vi "CodigoLabView 3.vi"() -> (11 "Releb 2":bool)   [LabVIEW 2025]
uses:
  <vilib>/Utility/NIReport.llb/Report Type.ctl
  <vilib>/Instr/_visa.llb/VISA Configure Serial Port (Instr).vi
  <vilib>/addons/_office/excel.llb/Excel Easy Table (str).vi
  <vilib>/Utility/NIReport.llb/NI_report.lvclass
  <vilib>/Utility/NIReport.llb/NI_ReportGenerationCore.lvlib
  <vilib>/addons/_office/NI_ReportGenerationToolkit.lvlib
  <vilib>/Utility/NIReport.llb/Excel/NI_Excel.lvclass
panel:
  out "Releb 4":bool
  out "Relea 4":bool
  out "Rele 4":bool
  out "Boolean 4":bool
  out "Estado 4":string
  in  "Relé N°4":bool
  out "Potencia 4":string
  out "Releb 3":bool
  out "Relea 3":bool
  out "Rele 3":bool
  out "Boolean 3":bool
  out "Estado 3":string
  out "Potencia 3":string
  in  "Relé N°3":bool
  out "Relea 2":bool
  out "Rele 2":bool
  out "Boolean 2":bool
  out "Estado 2":string
  out "Potencia 2":string
  in  "Relé N°2":bool
  out "Releb 1":bool
  out "Relea 1":bool
  out "Rele 1":bool
  out "Boolean":bool
  out "Estado 1":string
  out "Potencia 1":string
  in  "Relé N°1":bool
  in  "template (empty)":path
  out "Tensión":string
  in  "VISA resource name":refnum<visa-resource-name>
  in  "stop":bool
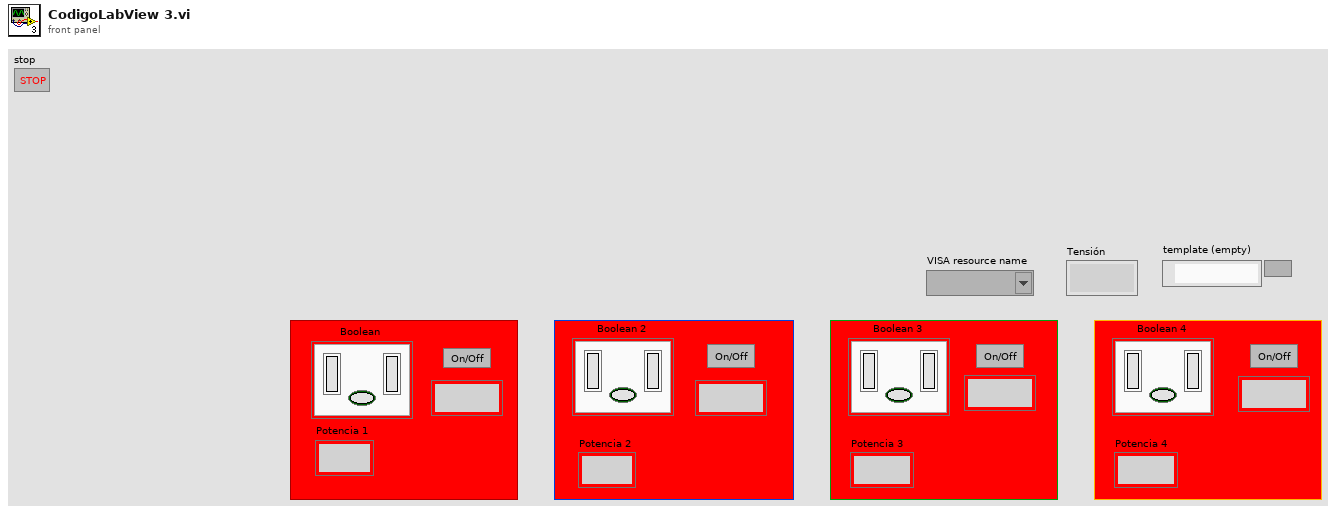
[diagram p1: front panel]
types:
  T1 = cluster{"W1":string, "W2":string, "W3":string, "W4":string, "V":string}
  T2 = typedef "NI_ReportGenerationCore.lvlib/Report Type.ctl" = enum16{"HTML", "Word", "Excel"}
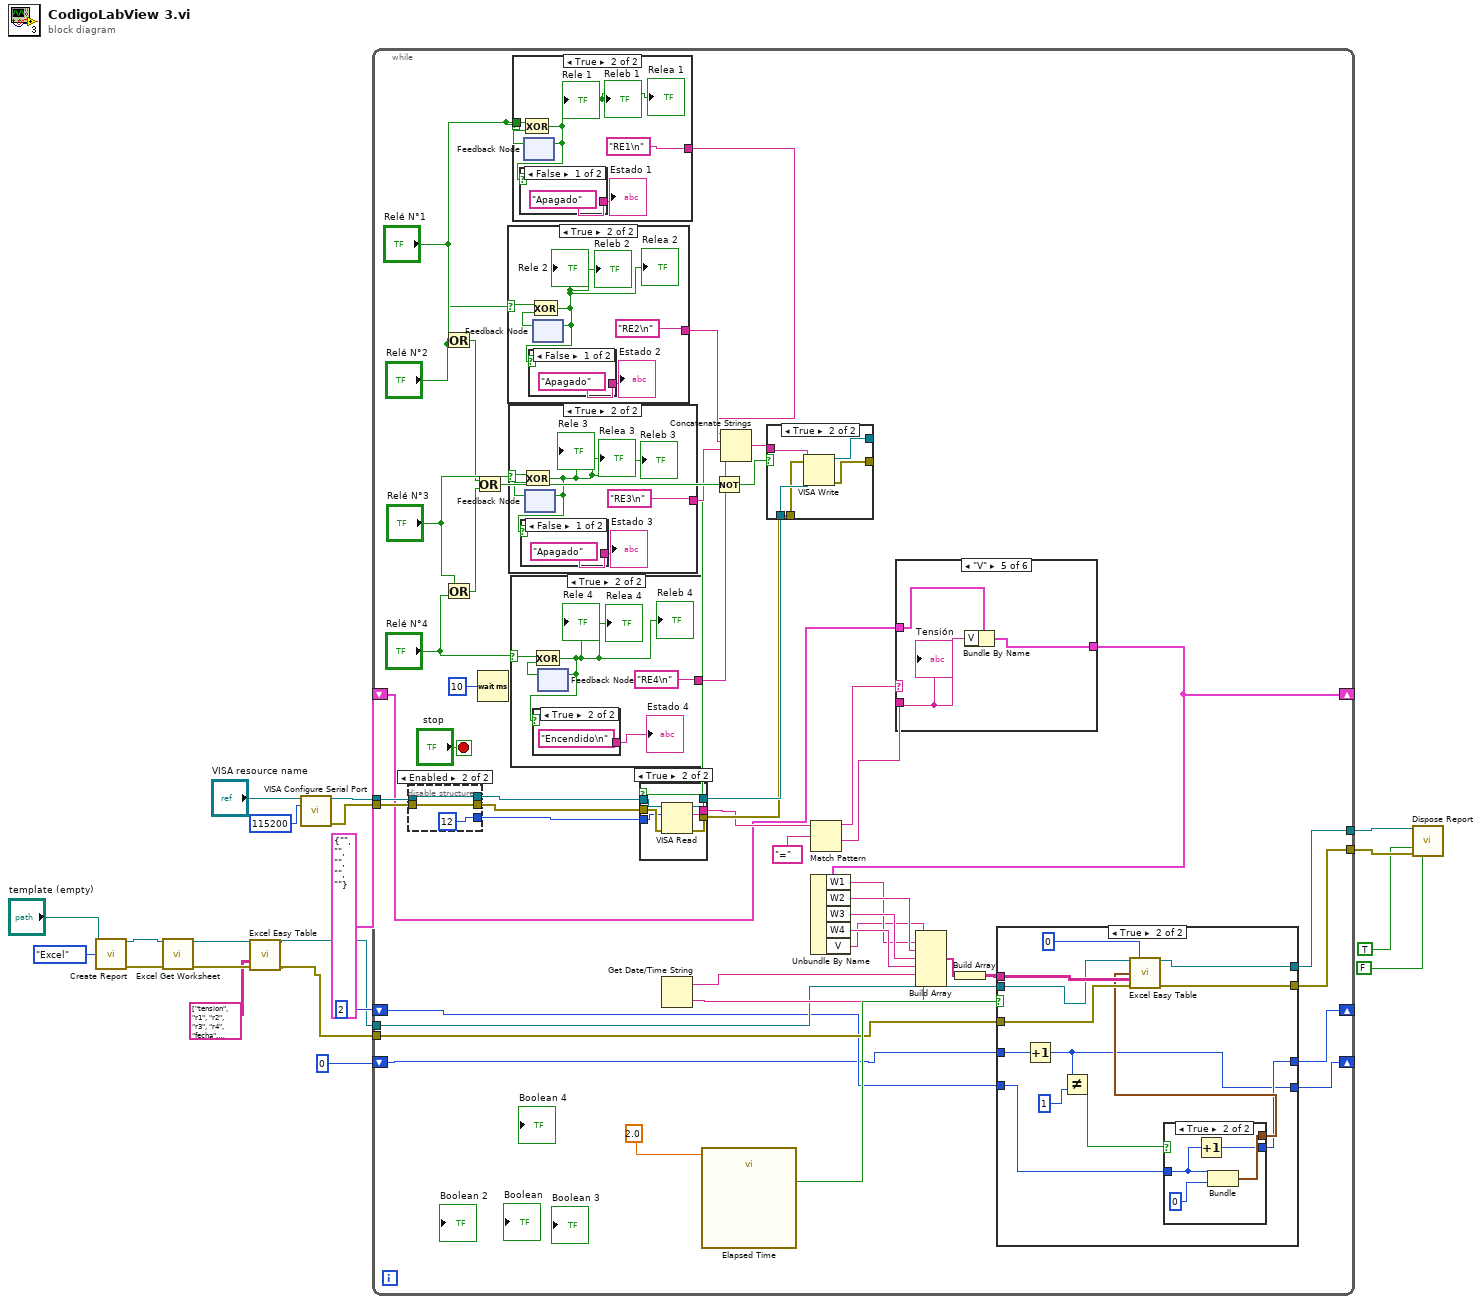
[diagram p0: block diagram]
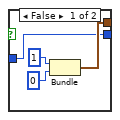
[diagram p3: hidden frame]
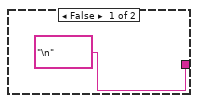
[diagram p4: hidden frame]
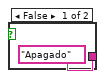
[diagram p5: hidden frame]
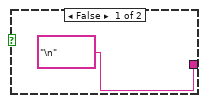
[diagram p6: hidden frame]
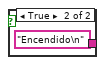
[diagram p7: hidden frame]
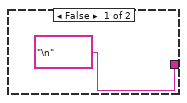
[diagram p8: hidden frame]
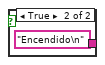
[diagram p9: hidden frame]
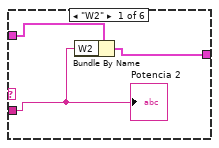
[diagram p10: hidden frame]
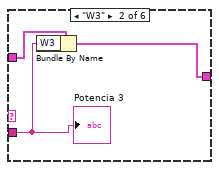
[diagram p11: hidden frame]
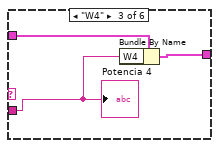
[diagram p12: hidden frame]
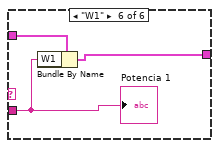
[diagram p14: hidden frame]
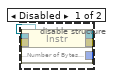
[diagram p15: hidden frame]
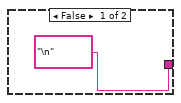
[diagram p18: hidden frame]
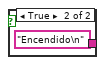
[diagram p19: hidden frame]
diagram:
  n1 = call <vilib>:"Create Report.vi"("report type"=Report_Type."Excel", "template (empty)"="template (empty)") -> ("report out"=w10:refnum<class "NI_report.lvclass">, "error out"=w9:errorcluster)  [unwired: 12 in]
  n2 = call <vilib>:"Excel Get Worksheet.vi"("report in"=w10, "error in (no error)"=w9) -> ("report out"=w4:refnum<class "NI_report.lvclass">, "error out"=w3:errorcluster)  [unwired: 12 in]
  n3 = call-poly <vilib>:"Excel Easy Table.vi"("report in"=w4, "text data"=string[][] [["tension", "r1", "r2", "r3", "r4", "fecha", "hora"]], "error in (no error)"=w3) -> ("report out"=w5:refnum<class "NI_report.lvclass">, "error out"=w6:errorcluster)  [unwired: 8 in, 3 out]
  n4 = call-poly "VISA Configure Serial Port"("VISA resource name"="VISA resource name", "baud rate (9600)"=u32 115200) -> ("VISA resource name out"=w20:refnum<visa-resource-name>, "error out"=w17:errorcluster)  [unwired: 12 in]
  n5 = while {
    tunnel: w20 -> [w66]
    tunnel: w17 -> [w65]
    tunnel: [w44] -> w14
    tunnel: [w43] -> w13
    tunnel: w5 -> [w37]
    tunnel: w6 -> [w36]
    shift-right: [w34] -> _
    shift-left: 2 -> [w35]
    shift-right: [w32] -> _
    shift-left: 0 -> [w33]
    shift-right: [w24] -> _
    shift-left: T1 {"W1"="", "W2"="", "W3"="", "W4"="", "V"=""} -> [w29]
    stop <- "stop" stop-if-true
    n6 = disable-structure shown="Enabled" {
      disable-tunnel: w66 -> [w137 w140]
      disable-tunnel: w65 -> [w136 w139]
      disable-tunnel: [w135 w140] -> w62
      disable-tunnel: [w134 u32 12 ("Bytes at Port")] -> w61
      disable-tunnel: [w133 w139] -> w60
      frame Disabled {
        n7 = property class="Instr"(reference=w137, error in=w136) -> (reference out=w135:refnum<visa-resource-name>, error out=w133:errorcluster, "Serial Settings:Number of Bytes at Serial Port"=w134:u32)
      }
      frame Enabled {
      }
    }
    n8 = Or(x="Relé N°1", y="Relé N°2") -> (x .or. y?=w51:bool)
    n9 = Or(x="Relé N°3", y="Relé N°4") -> (x .or. y?=w50:bool)
    n10 = Or(x=w51, y=w50) -> (x .or. y?=w55:bool)
    n11 = Wait (ms)(milliseconds to wait=u32 10) -> ()  [unwired: 1 out]
    n12 = case shown="True" "Relé N°2" {
      selector: "Relé N°2" -> [_ w111]
      tunnel: ["\n" "RE2\n"] -> w47
      frame False {
      }
      frame True {
        n13 = feedback #1() -> (w113:bool)  [unwired: 1 in]
        n14 = Exclusive Or(1:w113, 2:w111) -> (0:w110:bool)
        "Rele 2" <- w110
        "Releb 2" <- w110
        "Relea 2" <- w110
        n15 = case shown="False" w110 {
          tunnel: ["Apagado" "Encendido\n"] -> w112
          frame False {
          }
          frame True {
          }
        }
        "Estado 2" <- w112
        n16 = feedback-in #1(w110) -> ()
      }
    }
    n17 = case shown="True" "Relé N°3" {
      selector: "Relé N°3" -> [_ w103]
      tunnel: ["\n" "RE3\n"] -> w49
      frame False {
      }
      frame True {
        n18 = feedback #2() -> (w105:bool)  [unwired: 1 in]
        n19 = Exclusive Or(1:w105, 2:w103) -> (0:w102:bool)
        "Releb 3" <- w102
        "Relea 3" <- w102
        "Rele 3" <- w102
        n20 = case shown="False" w102 {
          tunnel: ["Apagado" "Encendido\n"] -> w104
          frame False {
          }
          frame True {
          }
        }
        "Estado 3" <- w104
        n21 = feedback-in #2(w102) -> ()
      }
    }
    n22 = case shown="True" "Relé N°4" {
      selector: "Relé N°4" -> [_ w95]
      tunnel: ["\n" "RE4\n"] -> w48
      frame False {
      }
      frame True {
        n23 = feedback #3() -> (w97:bool)  [unwired: 1 in]
        n24 = Exclusive Or(1:w97, 2:w95) -> (0:w94:bool)
        "Rele 4" <- w94
        "Releb 4" <- w94
        "Relea 4" <- w94
        n25 = case shown="True" w94 {
          tunnel: ["Apagado" "Encendido\n"] -> w96
          frame False {
          }
          frame True {
          }
        }
        "Estado 4" <- w96
        n26 = feedback-in #3(w94) -> ()
      }
    }
    n27 = case shown="True" "Relé N°1" {
      tunnel: ["\n" "RE1\n"] -> w21
      tunnel: "Relé N°1" -> [_ w160]
      frame False {
      }
      frame True {
        n28 = feedback #4() -> (w159:bool)  [unwired: 1 in]
        n29 = Exclusive Or(1:w159, 2:w160) -> (0:w157:bool)
        "Rele 1" <- w157
        "Relea 1" <- w157
        "Releb 1" <- w157
        n30 = case shown="False" w157 {
          tunnel: ["Apagado" "Encendido\n"] -> w158
          frame False {
          }
          frame True {
          }
        }
        "Estado 1" <- w158
        n31 = feedback-in #4(w157) -> ()
      }
    }
    n32 = Get Date/Time String() -> (date string=w39:string, time string=w38:string)  [unwired: 3 in]
    n33 = call "Elapsed Time"("Time Target (s)"=2.0) -> ("Time has Elapsed"=w40:bool)  [unwired: 11 in, 7 out]
    n34 = Not(x=w55) -> (.not. x?=w42:bool)
    n35 = case shown="True" w42 {
      tunnel: [w142 w148] -> w64
      tunnel: [w141 w147] -> w63
      tunnel: w60 -> [w141 w146]
      tunnel: w62 -> [w142 w145]
      tunnel: w61 -> [_ w144]
      tunnel: [_ w143] -> w31
      frame False {
      }
      frame True {
        n36 = VISA Read(VISA resource name=w145, byte count=w144, error in (no error)=w146) -> (VISA resource name out=w148:refnum<visa-resource-name>, read buffer=w143:string, error out=w147:errorcluster)  [unwired: 1 out]
      }
    }
    n37 = Concatenate Strings(w21, w47, w49, w48) -> (w22:string)
    n38 = case shown="True" w55 {
      tunnel: [w150 w155] -> _
      tunnel: [w149 w154] -> _
      tunnel: w64 -> [w150 w153]
      tunnel: w63 -> [w149 w152]
      tunnel: w22 -> [_ w151]
      frame False {
      }
      frame True {
        n39 = VISA Write(VISA resource name=w153, write buffer=w151, error in (no error)=w152) -> (VISA resource name out=w155:refnum<visa-resource-name>, error out=w154:errorcluster)  [unwired: 1 out]
      }
    }
    n40 = Match Pattern(string=w31, regular expression="=") -> (before substring=w57:string, after substring=w30:string)  [unwired: 1 in, 2 out]
    n41 = case shown="\"V\"" w57 {
      tunnel: w30 -> [w118 w121 w123 _ w127 w131]
      tunnel: w29 -> [w119 w122 w124 w126 w129 w132]
      tunnel: [w117 w120 w125 w126 w128 w130] -> w24
      frame "W2" {
        n42 = Bundle By Name(cluster=w119, "W2"=w118) -> (w117:T1)
        "Potencia 2" <- w118
      }
      frame "W3" {
        n43 = Bundle By Name(cluster=w122, "W3"=w121) -> (w120:T1)
        "Potencia 3" <- w121
      }
      frame "W4" {
        n44 = Bundle By Name(cluster=w124, "W4"=w123) -> (w125:T1)
        "Potencia 4" <- w123
      }
      frame "False", Default {
      }
      frame "V" {
        n45 = Bundle By Name(cluster=w129, "V"=w127) -> (w128:T1)
        "Tensión" <- w127
      }
      frame "W1" {
        n46 = Bundle By Name(cluster=w132, "W1"=w131) -> (w130:T1)
        "Potencia 1" <- w131
      }
    }
    n47 = Unbundle By Name(w24) -> ("W1"=w25:string, "W2"=w26:string, "W3"=w27:string, "W4"=w28:string, "V"=w23:string)
    n48 = Build Array(w23, w25, w26, w27, w28, w39, w38) -> (w46:string[])
    n49 = Build Array(w46) -> (w45:string[][])
    n50 = case shown="True" w40 {
      tunnel: w45 -> [_ w84]
      tunnel: w36 -> [w71 w83]
      tunnel: [w70 w82] -> w44
      tunnel: [w71 w81] -> w43
      tunnel: w37 -> [w70 w80]
      tunnel: w35 -> [w69 w77]
      tunnel: [w69 w76] -> w34
      tunnel: w33 -> [w68 w75]
      tunnel: [w68 w72] -> w32
      frame False {
      }
      frame True {
        n51 = Increment(x=w75) -> (x+1=w72:i32)
        n52 = Not Equal?(x=w72, y=1) -> (x != y?=w73:bool)
        n53 = case shown="True" w73 {
          tunnel: [w86 w92] -> w79
          tunnel: w77 -> [w85 w90]
          tunnel: [w85 w89] -> w76
          frame False {
            n54 = Bundle(1, 0) -> (w86:cluster{i32, i32})  [unwired: 1 in]
          }
          frame True {
            n55 = Increment(x=w90) -> (x+1=w89:i32)
            n56 = Bundle(w90, 0) -> (w92:cluster{i32, i32})  [unwired: 1 in]
          }
        }
        n57 = call-poly <vilib>:"Excel Easy Table.vi"("report in"=w80, "iteration"=0, "start (0, 0)"=w79, "text data"=w84, "error in (no error)"=w83) -> ("report out"=w82:refnum<class "NI_report.lvclass">, "error out"=w81:errorcluster)  [unwired: 6 in, 3 out]
      }
    }
  }
  n58 = call-dynamic "Dispose Report.vi"("report in"=w14, "save changes? (F)"=TRUE, "error in (no error)"=w13, "close report? (T)"=FALSE) -> ()  [unwired: 11 in, 1 out]
